vi "rs232_string_params_to_ring.vi"(9 "flow control string":string, 10 "parity string":string, 11 "baud rate string":string) -> (1 "Flow control":u16(ring) items=["None", "XON/XOFF", "RTS/CTS", "XON/XOFF & RTS/CTS", "DTR/DSR", "XON/XOFF & DTR/DSR"], 2 "Parity":enum16{"None", "Odd", "Even", "Mark", "Space"}(ring), 3 "Baud rate":u32)   [LabVIEW 2015]
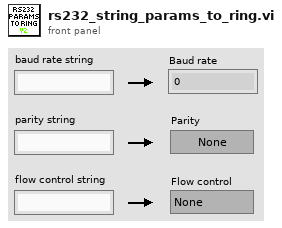
[diagram p1: front panel]
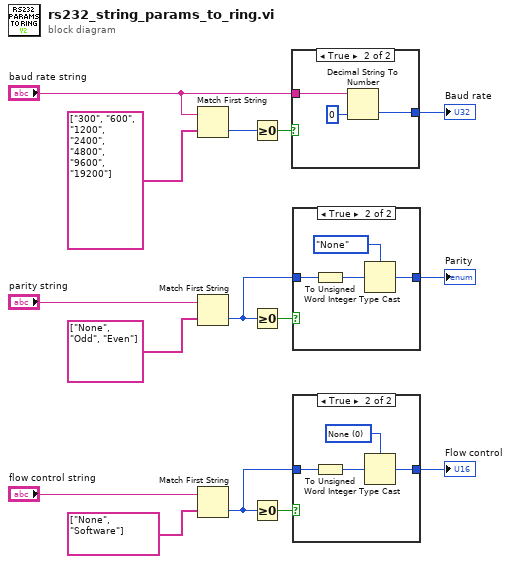
[diagram p0: block diagram]
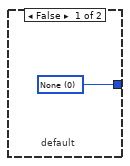
[diagram p2: hidden frame]
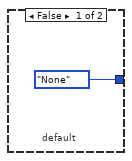
[diagram p3: hidden frame]
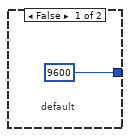
[diagram p4: hidden frame]
diagram:
  n1 = Match First String(2:string[] ["300", "600", "1200", "2400", "4800", "9600", "19200"] ("string array"), 3:"baud rate string") -> (0:w14:i32)  [unwired: 1 out]
  n2 = Match First String(2:string[] ["None", "Odd", "Even"] ("string array"), 3:"parity string") -> (0:w7:i32)  [unwired: 1 out]
  n3 = Match First String(2:string[] ["None", "Software"] ("string array"), 3:"flow control string") -> (0:w6:i32)  [unwired: 1 out]
  n4 = Greater Or Equal To 0?(x=w14) -> (x >= 0?=w11:bool)
  n5 = Greater Or Equal To 0?(x=w7) -> (x >= 0?=w9:bool)
  n6 = Greater Or Equal To 0?(x=w6) -> (x >= 0?=w4:bool)
  n7 = case shown="True" w11 {
    tunnel: "baud rate string" -> [_ w19]
    tunnel: [u32 9600 w18] -> w12
    frame False {
      # "default"
    }
    frame True {
      n8 = Decimal String To Number(string=w19, default (0L)=u32 0 ("default (0 I32)")) -> (number=w18:u32)  [unwired: 1 in, 1 out]
    }
  }
  "Baud rate" <- w12
  n9 = case shown="True" w9 {
    tunnel: [enum16{"None", "Odd", "Even", "Mark", "Space"}."None" ("parity (0:none)") w24] -> w1
    tunnel: w7 -> [_ w23]
    frame False {
      # "default"
    }
    frame True {
      n10 = To Unsigned Word Integer(number=w23) -> (unsigned 16bit integer=w22:u16)
      n11 = Type Cast(type=enum16{"None", "Odd", "Even", "Mark", "Space"}."None" ("parity (0:none)"), x=w22) -> (*(type *) &x=w24:enum16{"None", "Odd", "Even", "Mark", "Space"})
    }
  }
  "Parity" <- w1
  n12 = case shown="True" w4 {
    tunnel: [w25 w29] -> w2
    tunnel: w6 -> [_ w28]
    frame False {
      w25 = u16 0 items=["None", "XON/XOFF", "RTS/CTS", "XON/XOFF & RTS/CTS", "DTR/DSR", "XON/XOFF & DTR/DSR"] ("flow control (0:none)")
      # "default"
    }
    frame True {
      w26 = u16 0 items=["None", "XON/XOFF", "RTS/CTS", "XON/XOFF & RTS/CTS", "DTR/DSR", "XON/XOFF & DTR/DSR"] ("flow control (0:none)")
      n13 = To Unsigned Word Integer(number=w28) -> (unsigned 16bit integer=w27:u16)
      n14 = Type Cast(type=w26, x=w27) -> (*(type *) &x=w29:u16)
    }
  }
  "Flow control" <- w2
